vi "Destroy.vi"(0 "reference":refnum<class "VdTcpIP.lvclass">, 5 "error in (no error)":errorcluster) -> (19 "error out":errorcluster)   [LabVIEW 2020, in "VdTcpIP.lvclass"]
doc: "Destroys an object created with a VdSocket constructor VI or a subclass of the VdSocket class. This VI must be reentrant.\n\n[GOOP 2.0.11]"
uses:
  VdTcpIP.lvclass
panel:
  out "reference out":refnum<class "VdTcpIP.lvclass">
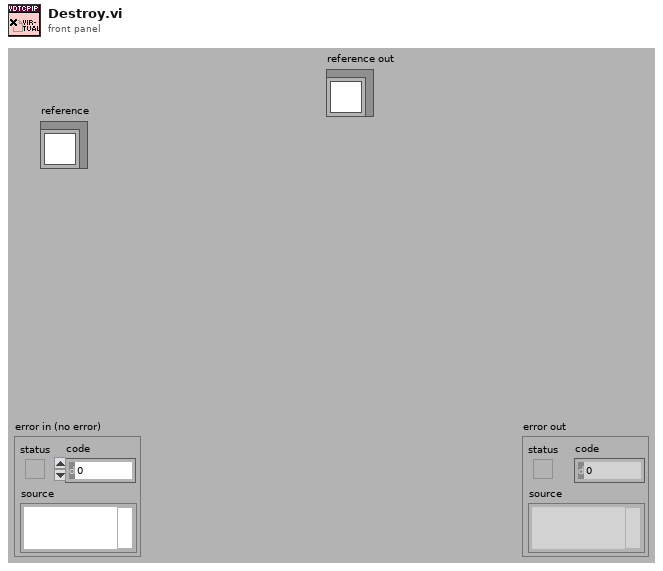
[diagram p1: front panel]
types:
  T1 = typedef "VdTcpIP.lvclass/ObjectAttributes.ctl" = cluster{"IP-Address":string, "Port":u16, "Connection":refnum<k5>, "Listener":refnum<k5>, "ListenerConnection":refnum<k5>, "Listner":bool, "ListnerProcessRunning":bool, "InConnections":refnum<k5>[], "InConnectionsIP":string[], "InConnectionAdded":refnum<notifier>, "RunVIOnNewConnection":variant, "DataToNewConnectionVI":cluster{"ControlName":string, "ControlValue":variant}[], "WebServicesURL_Location(http://...)":string, "WebServicesPostWebPage(*.asmx)":string, "Semaphore":T2, "AutoReConnectTimes":i32, "AutoReConnectInterval(ms)":i32, "ConnectionTimeout":i32}
  T2 = typedef "Semaphore RefNum" = refnum<k1>
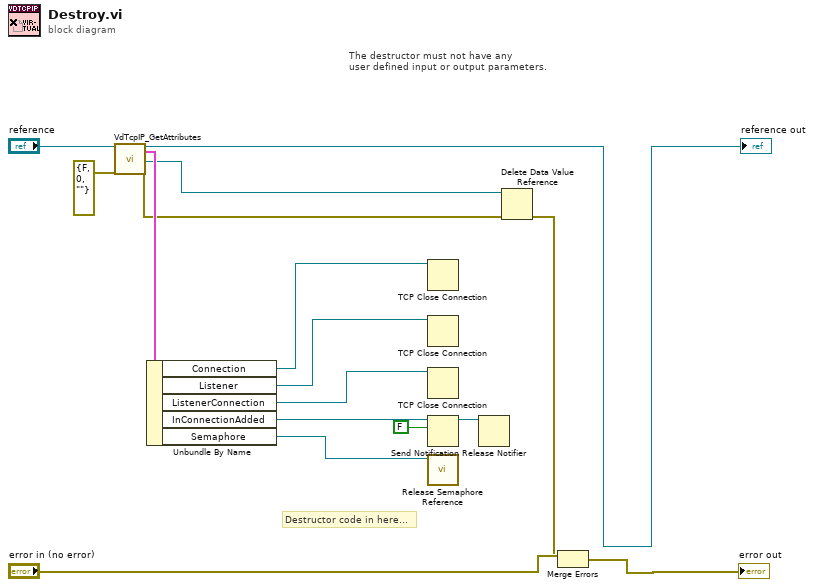
[diagram p0: block diagram]
diagram:
  # "Destructor code in here..."
  # "The destructor must not have any\nuser defined input or output parameters."
  n1 = call "VdTcpIP_GetAttributes.vi"("reference in"="reference", "error in (no error)"=errorcluster {"status"=FALSE, "code"=0, "source"=""}) -> ("reference out"=→"reference out":refnum<class "VdTcpIP.lvclass">, "Data"=w4:T1, "DataRef"=w3:refnum<data-value>, "error out"=w1:errorcluster)  [unwired: 1 in, 13 out]
  n2 = Unbundle By Name(w4) -> ("Connection"=w10:refnum<k5>, "Listener"=w9:refnum<k5>, "ListenerConnection"=w8:refnum<k5>, "InConnectionAdded"=w13:refnum<notifier>, "Semaphore"=w5:T2)
  n3 = TCP Close Connection(connection ID=w10) -> ()  [unwired: 1 in, 3 out]
  n4 = TCP Close Connection(connection ID=w9) -> ()  [unwired: 1 in, 3 out]
  n5 = TCP Close Connection(connection ID=w8) -> ()  [unwired: 1 in, 3 out]
  n6 = Send Notification(notification=FALSE, notifier=w13) -> (notifier out=w6:refnum<notifier>)  [unwired: 1 in, 1 out]
  n7 = call <vilib>:"Release Semaphore Reference.vi"("semaphore"=w5) -> ()  [unwired: 9 in, 2 out]
  n8 = Release Notifier(notifier=w6) -> ()  [unwired: 1 in, 4 out]
  n9 = Delete Data Value Reference(data value reference=w3, error in=w1) -> (error out=w2:errorcluster)  [unwired: 1 out]
  n10 = Merge Errors("error in (no error)", w2) -> (→"error out":errorcluster)
